vi "http check to close connection.vi"(11 "application request":T1) -> (1 "leave connection open?":bool, 2 "stop process?":bool, 3 "application request out":T1)   [LabVIEW 2016, in "Basic HTTP server.lvclass"]
uses:
  Basic HTTP server.lvclass
  http response.ctl
  http response packet type.ctl
  http header data.ctl
  headers/http headers.lvlib
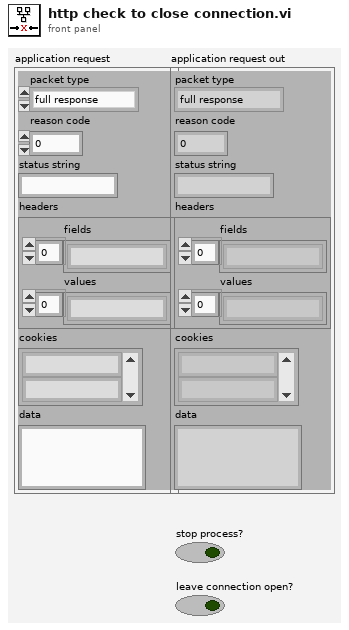
[diagram p1: front panel]
types:
  T1 = typedef "Basic HTTP server.lvclass/http response.ctl" = cluster{"packet type":T2, "reason code":u16, "status string":string, "headers":T3, "cookies":string[], "data":string}
  T2 = typedef "Basic HTTP server.lvclass/http response packet type.ctl" = enum16{"full response", "header only", "data only", "last data"}
  T3 = typedef "http headers.lvlib/http header data.ctl" = cluster{"fields":string[], "values":string[]}
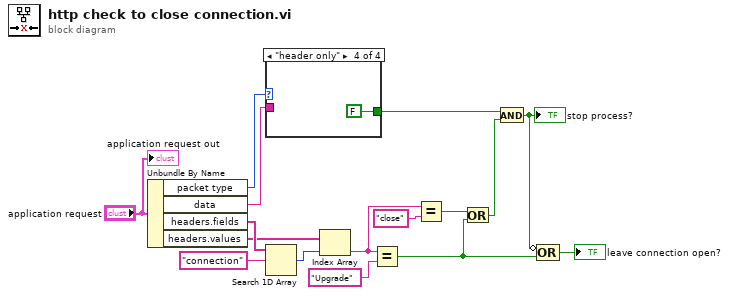
[diagram p0: block diagram]
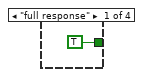
[diagram p2: hidden frame]
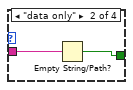
[diagram p3: hidden frame]
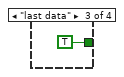
[diagram p4: hidden frame]
diagram:
  n1 = Unbundle By Name("application request") -> ("packet type"=w15:T2, "data"=w13:string, "headers.fields"=w8:string[], "headers.values"=w5:string[])
  n2 = case shown="\"header only\"" w15 {
    tunnel: [TRUE w18 TRUE FALSE] -> w14
    tunnel: w13 -> [_ w19 _ _]
    frame "full response" {
    }
    frame "data only" {
      n3 = Empty String/Path?(string/path=w19) -> (empty?=w18:bool)
    }
    frame "last data" {
    }
    frame "header only" {
    }
  }
  n4 = Search 1D Array(1D array=w8, element="connection" ("name")) -> (index of element=w6:i32)  [unwired: 1 in]
  n5 = Index Array(array=w5, index=w6) -> (element=w4:string)
  n6 = Equal?(x=w4, y="Upgrade" ("name")) -> (x = y?=w9:bool)
  n7 = Equal?(x=w4, y="close" ("name")) -> (x = y?=w3:bool)
  n8 = Or(x=w3, y=w9) -> (x .or. y?=w10:bool)
  n9 = And(x=w14, y=w10) -> (x .and. y?=w12:bool)
  "stop process?" <- w12
  n10 = Compound Arithmetic op=OR(invert w12, w9) -> (→"leave connection open?":bool)
  "application request out" <- "application request"
